vi "Write EtherCAT.vi"(8 "error in (no error)":errorcluster, 10 "EtherCAT?":bool, 11 "RSI Module in":refnum<class "RSI Module.lvclass">) -> (0 "error out":errorcluster, 3 "RSI Module out":refnum<class "RSI Module.lvclass">)   [LabVIEW 2020, in "Modules.lvlib" / "RSI Module.lvclass"]
uses:
  RSI Module.lvclass
  RSI Module.lvclass/RSI Module.ctl
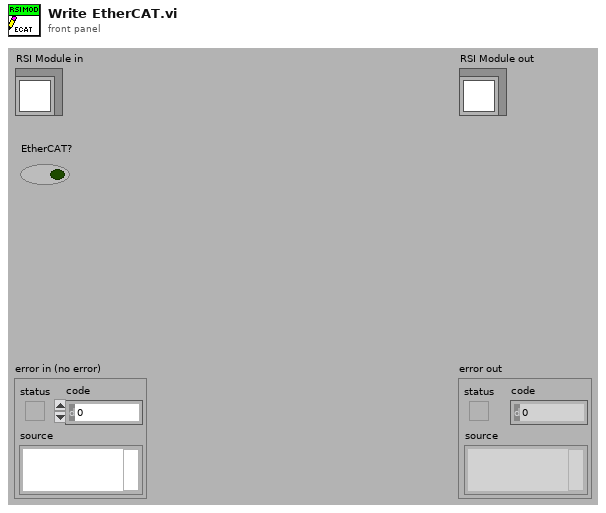
[diagram p1: front panel]
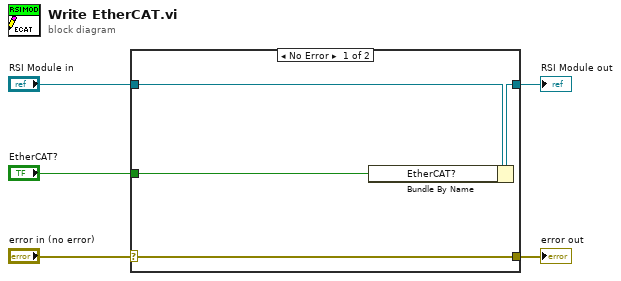
[diagram p0: block diagram]
diagram:
  n1 = case shown="No Error" "error in (no error)" {
    selector: "error in (no error)" -> [w9 w10]
    tunnel: [w9 w10] -> w4
    tunnel: [w7 w11] -> w2
    tunnel: "RSI Module in" -> [w8 w11]
    tunnel: "EtherCAT?" -> [w6 _]
    frame No Error {
      n2 = Bundle By Name(cluster=w8, "EtherCAT?"=w6) -> (w7:refnum<class "RSI Module.lvclass">)
    }
    frame Error {
    }
  }
  "error out" <- w4
  "RSI Module out" <- w2
